vi "getSpeedAndGainSettings.vi"(6 "Delay between send and receive [ms]":i32=100, 8 "error in (no error)":errorcluster, 11 "CCD in":refnum<class "CCD.lvclass">) -> (0 "error out":errorcluster, 1 "CCD-gain options":T3, 2 "CCD-speeds options":T1, 3 "CCD out":refnum<class "CCD.lvclass">)   [LabVIEW 2023, in "CCD.lvclass"]
uses:
  CCD.lvclass
  GainsArray.ctl
  Gain.ctl
  SpeedsArray.ctl
  Speed.ctl
  20f7d3bd-08ac-4524-9bed-df36c1da25a0.vi
  a21955fc-e3a0-4e36-8495-41f1bfac7860.vi
  1c95c044-04a3-4674-b8b9-390d512e0141.vi
  <vilib>/JDP Science/JSONtext/Next JSON Value.vi
  <vilib>/JDP Science/JSONtext/String Subset.vi
  <vilib>/JDP Science/JSONtext/Parsing/Advance past next JSON Value (inlined COPY).vi
  <vilib>/JDP Science/JSONtext/Parsing/Advance past whitespace.vi
  <vilib>/JDP Science/JSONtext/Parsing/Advance past String.vi
  <vilib>/JDP Science/JSONtext/Parsing/Advance past Number.vi
  <vilib>/JDP Science/JSONtext/Parsing/Advance past Line Ending.vi
  <vilib>/JDP Science/JSONtext/Variant to JSON Text.vi
  <vilib>/JDP Science/JSONtext/Set Item.vi
  <vilib>/JDP Science/JSONtext/Parsing/Parse Full Path or Item Name.vi
  <vilib>/JDP Science/JSONtext/Parsing/Advance past Array.vi
  <vilib>/JDP Science/JSONtext/Parsing/Advance past Object.vi
  <vilib>/JDP Science/JSONtext/support/Error Cluster From Code.vi
  <vilib>/JDP Science/JSONtext/Offset/Find Item Locations by Path.vi
  <vilib>/JDP Science/JSONtext/JSON text to Variant.vi
  <vilib>/JDP Science/JSONtext/LVClass Serializer/JSONtext LVClass Serializer.lvclass
  GenericDevice/GenericDevice.lvclass
  <vilib>/IlluminatedG/lv-web-crypto/lv-json/JSON/JSON.lvlib
  <vilib>/JDP Science/JSONtext/JSONtext.lvlib
panel:
  # "Connector Pane"
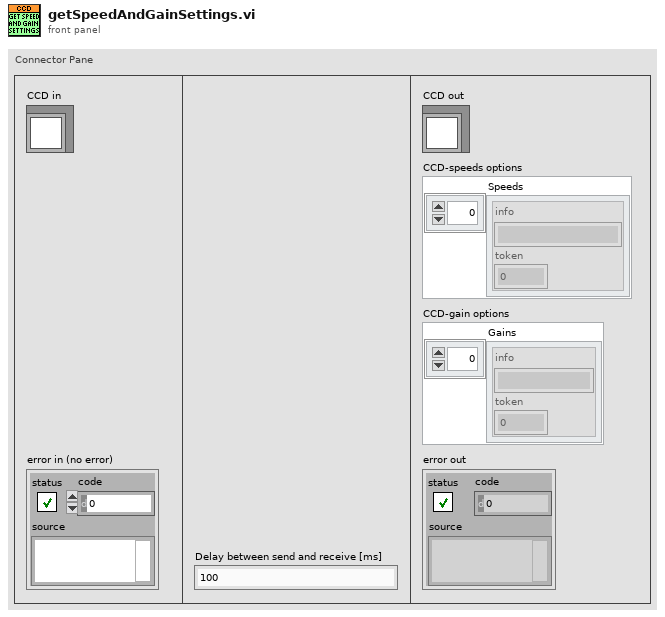
[diagram p1: front panel]
types:
  T1 = typedef "CCD.lvclass/SpeedsArray.ctl" = cluster{"Speeds":T2[]}
  T2 = typedef "CCD.lvclass/Speed.ctl" = cluster{"info":string, "token":u16}
  T3 = typedef "CCD.lvclass/GainsArray.ctl" = cluster{"Gains":T4[]}
  T4 = typedef "CCD.lvclass/Gain.ctl" = cluster{"info":string, "token":u16}
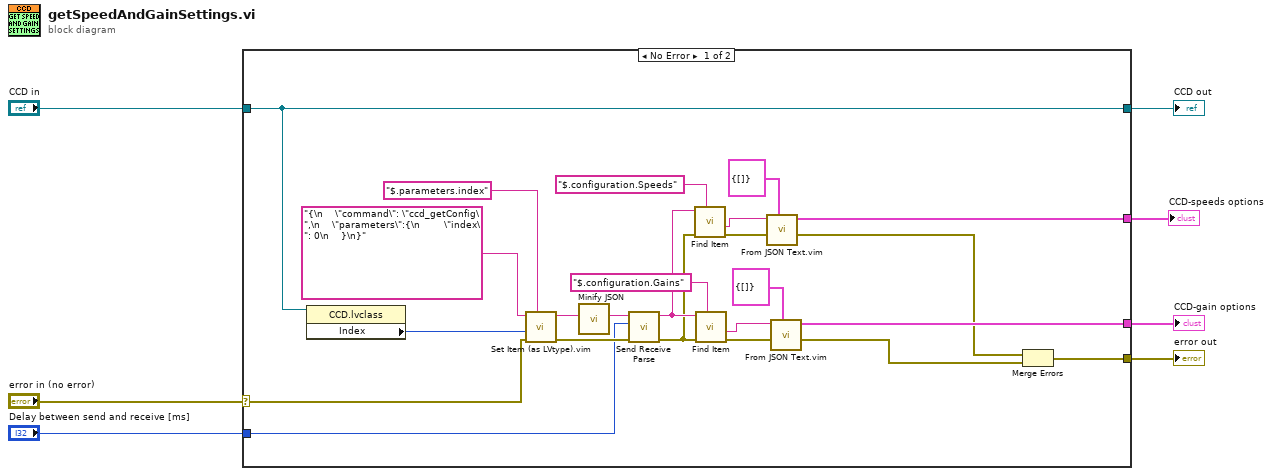
[diagram p0: block diagram]
diagram:
  n1 = case shown="No Error" "error in (no error)" {
    selector: "error in (no error)" -> [w27 w33]
    tunnel: [w13 w33] -> w6
    tunnel: [w29 w32] -> w4
    tunnel: "CCD in" -> [w29 w32]
    tunnel: [w26 _] -> w2
    tunnel: "Delay between send and receive [ms]" -> [w22 _]
    tunnel: [w8 _] -> w1
    frame No Error {
      n2 = property class="CCD.lvclass"(reference=w29) -> ("Index"=w28:i32)  [unwired: 1 in, 2 out]
      n3 = call "Set Item (as LVtype).vim"("$Path or Item Name"="$.parameters.index", "error in (no error)"=w27, "Anything"=w28, "JSON"="{\n    \"command\": \"ccd_getConfig\",\n    \"parameters\":{\n        \"index\": 0\n    }\n}") -> ("error out"=w25:errorcluster, "<JSON>"=w24:string)  [unwired: 4 in, 1 out]
      n4 = call <vilib>:"Minify JSON.vi"("JSON String"=w24) -> ("Minified JSON"=w23:string)  [unwired: 10 in]
      n5 = call "Send Receive Parse.vi"("error in"=w25, "Delay between send and receive [ms]"=w22, "<JSON>"=w23) -> ("error out"=w15:errorcluster, "results-JSON string"=w16:string)  [unwired: 6 in, 1 out]
      n6 = call <vilib>:"Find Item.vi"("$Path or Item Name"="$.configuration.Speeds", "error in (no error)"=w15, "JSON"=w16) -> ("error out"=w11:errorcluster, "<JSON>"=w12:string)  [unwired: 5 in, 2 out]
      n7 = call <vilib>:"Find Item.vi"("$Path or Item Name"="$.configuration.Gains", "error in (no error)"=w15, "JSON"=w16) -> ("error out"=w21:errorcluster, "<JSON>"=w20:string)  [unwired: 5 in, 2 out]
      n8 = call "From JSON Text.vim"("Data Type and Default Value"=T1 {"Speeds"=[]} ("speeds array"), "error in (no error)"=w11, "JSON"=w12) -> ("error out"=w9:errorcluster, "Data out"=w8:T1)  [unwired: 7 in]
      n9 = call "From JSON Text.vim"("Data Type and Default Value"=T3 {"Gains"=[]} ("gains array"), "error in (no error)"=w21, "JSON"=w20) -> ("error out"=w14:errorcluster, "Data out"=w26:T3)  [unwired: 7 in]
      n10 = Merge Errors(w9, w14) -> (w13:errorcluster)
    }
    frame Error {
    }
  }
  "error out" <- w6
  "CCD out" <- w4
  "CCD-gain options" <- w2
  "CCD-speeds options" <- w1
